vi "PathPlanner_PathFinder_DoReset.vi"   [LabVIEW 2019, in "PathPlanner24.lvlib"]
uses:
  PathPlanner24.lvlib
  PathPlanner_GridPosition_Get.vi
  PathPlanner_PathFinder_Heuristic.vi
  PathPlanner_PathFinder_Globals.vi
types:
  T1 = typedef "PathPlanner24.lvlib/PathPlannerFinderGridPosition.ctl" = cluster{"X":i32, "Y":i32}
  T2 = typedef "PathPlanner24.lvlib/PathPlannerFinderDoublePair.ctl" = cluster{"A":dbl, "B":dbl}
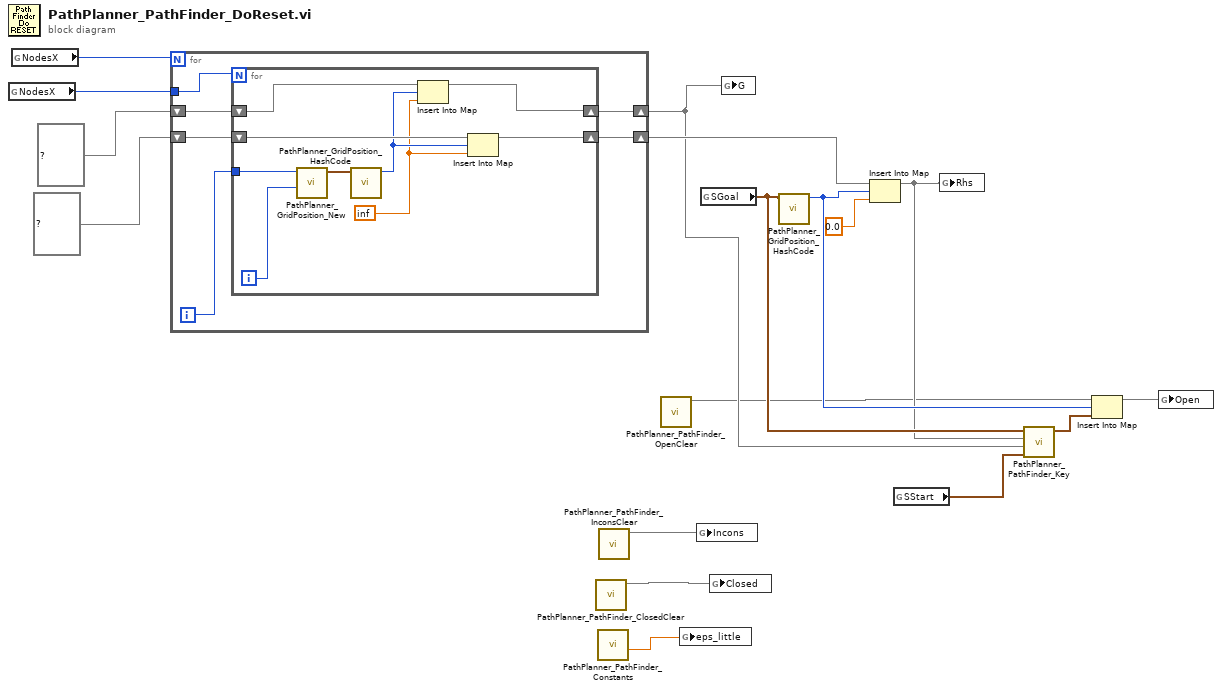
[diagram p0: block diagram]
diagram:
  n1 = global read "PathPlanner_PathFinder_Globals.vi" "NodesX"() -> (w16:i32)
  n2 = global read "PathPlanner_PathFinder_Globals.vi" "NodesX"() -> (w17:i32)
  n3 = for {
    N: w17 -> [_]
    tunnel: w16 -> [w23]
    shift-right: [w19] -> w5
    shift-left: map{i32, dbl} {} ("G") -> [w22]
    shift-right: [w18] -> w13
    shift-left: map{i32, dbl} {} ("Rhs") -> [w20]
    i -> [w21]
    n4 = for {
      N: w23 -> [_]
      shift-right: [w25] -> w19
      shift-left: w22 -> [w32]
      tunnel: w21 -> [w31]
      shift-right: [w24] -> w18
      shift-left: w20 -> [w28]
      i -> [w30]
      w26 = inf
      n5 = call "PathPlanner_GridPosition_New.vi"("Y"=w30, "X"=w31) -> ("GridPosition"=w29:T1)  [unwired: 9 in]
      n6 = call "PathPlanner_GridPosition_HashCode.vi"("GridPosition"=w29) -> ("HashCode"=w27:i32)  [unwired: 10 in]
      n7 = Insert Into Map(map in=w32, key=w27, value=w26) -> (map out=w25:map{i32, dbl})  [unwired: 2 out]
      n8 = Insert Into Map(map in=w28, key=w27, value=w26) -> (map out=w24:map{i32, dbl})  [unwired: 2 out]
    }
  }
  n9 = call "PathPlanner_PathFinder_ClosedClear.vi"() -> ("Closed"=w1:set{T1})  [unwired: 11 in]
  n10 = call "PathPlanner_PathFinder_Constants.vi"() -> ("EPS"=w11:dbl)  [unwired: 9 in, 2 out]
  n11 = call "PathPlanner_PathFinder_InconsClear.vi"() -> ("Incons"=w2:map{i32, T2})  [unwired: 11 in]
  n12 = call "PathPlanner_PathFinder_OpenClear.vi"() -> ("Open"=w3:map{i32, T2})  [unwired: 11 in]
  n13 = global write "PathPlanner_PathFinder_Globals.vi" "eps_little"(w11) -> ()
  n14 = global write "PathPlanner_PathFinder_Globals.vi" "Incons"(w2) -> ()
  n15 = global read "PathPlanner_PathFinder_Globals.vi" "SGoal"() -> (w7:T1)
  n16 = global write "PathPlanner_PathFinder_Globals.vi" "Closed"(w1) -> ()
  n17 = global write "PathPlanner_PathFinder_Globals.vi" "G"(w5) -> ()
  n18 = call "PathPlanner_GridPosition_HashCode.vi"("GridPosition"=w7) -> ("HashCode"=w9:i32)  [unwired: 10 in]
  n19 = Insert Into Map(map in=w13, key=w9, value=0.0) -> (map out=w6:map{i32, dbl})  [unwired: 2 out]
  n20 = global read "PathPlanner_PathFinder_Globals.vi" "SStart"() -> (w4:T1)
  n21 = global write "PathPlanner_PathFinder_Globals.vi" "Rhs"(w6) -> ()
  n22 = call "PathPlanner_PathFinder_Key.vi"("Sstart"=w4, "G"=w5, "RHS"=w6, "S"=w7) -> ("DoublePair"=w8:T2)  [unwired: 7 in]
  n23 = Insert Into Map(map in=w3, key=w9, value=w8) -> (map out=w10:map{i32, T2})  [unwired: 2 out]
  n24 = global write "PathPlanner_PathFinder_Globals.vi" "Open"(w10) -> ()
